vi "SDT_WriteFileDecayCurves.vi"(4 "adc_re[dig]":i16=256, 5 "ActiveModule":string[](array[string]), 6 "EndTimeArray":dbl[](array[numeric]), 7 "DecayMatrix":u32[][](array[numeric]), 8 "ErrorIn":errorcluster, 9 "SPCdata":T13[](array[typedef]) {"scan_flyback" format="%x"}, 10 "FileType":T1=2 items=["non-Fifo"=1, "Fifo"=2, "FifoImage"=3], 11 "SDT-FilePath":path=path "\\\\lab13\\C/Users/jannis/Desktop/ZeissFifo.sdt") -> (0 "ErrorOut":errorcluster)   [LabVIEW 2019]
doc: "This VI writes a SDT-file to disc. The SetUp and the MeasureInfo blocks are created and appended with the data blocks. \nThis VI is limited to writing a DecayMatrix from a FIFO-Image recording and optional an IntensityImage to file. For single mode recordings use the spcmdll VI \\Public\\Configure\\Memory Transfer\\SPC_save_data_to_sdtfile.vi.\nFor a description of the format for the Data input cluster to this VI see the usage in \\Example\\ImagingEventStream-SimpleFifoImage.vi. Leave either of the cluster input arrays empty to not save them to disc.\nFor a description of the *.sdt file format see: SPC_data_file_structure.h\n\ninfo@becker-hickl.com"
uses:
  SPC_Controls/bhfile_header.ctl
  SPC_Controls/SPCdata.ctl
  SPC_Controls/MeasureInfo_PartB.ctl
  SPC_Controls/MeasStopInfo.ctl
  SPC_Controls/MeasFCSInfo.ctl
  SPC_Controls/MeasureInfo_PartE.ctl
  SPC_Controls/MeasHISTInfo.ctl
  SPC_Controls/HISTInfoExt.ctl
  SPC_Controls/MeasureInfo_PartI.ctl
  SPC_Controls/MeasureInfo_PartK.ctl
  SPC_Controls/MeasureInfo_PartM.ctl
  SPC_Controls/MeasureInfo.ctl
  SPC_Controls/BHFileBlockHeader.ctl
  SPC_Controls/FileType.ctl
panel:
  out "Info Block":string
  out "BHFileBlockHeaders":T2[](array[typedef])
  out "MeasureInfos":T3[](array[typedef]) {"MeasFCSInfo"."end_time" format="%#_7g"; "MeasStopInfo"."flags" format="x%x"}
  out "BlockLengths":i32[](array[numeric])
  out "bhfile_header":T14 {"chksum" format="x%x"; "header_valid" format="x%x"}
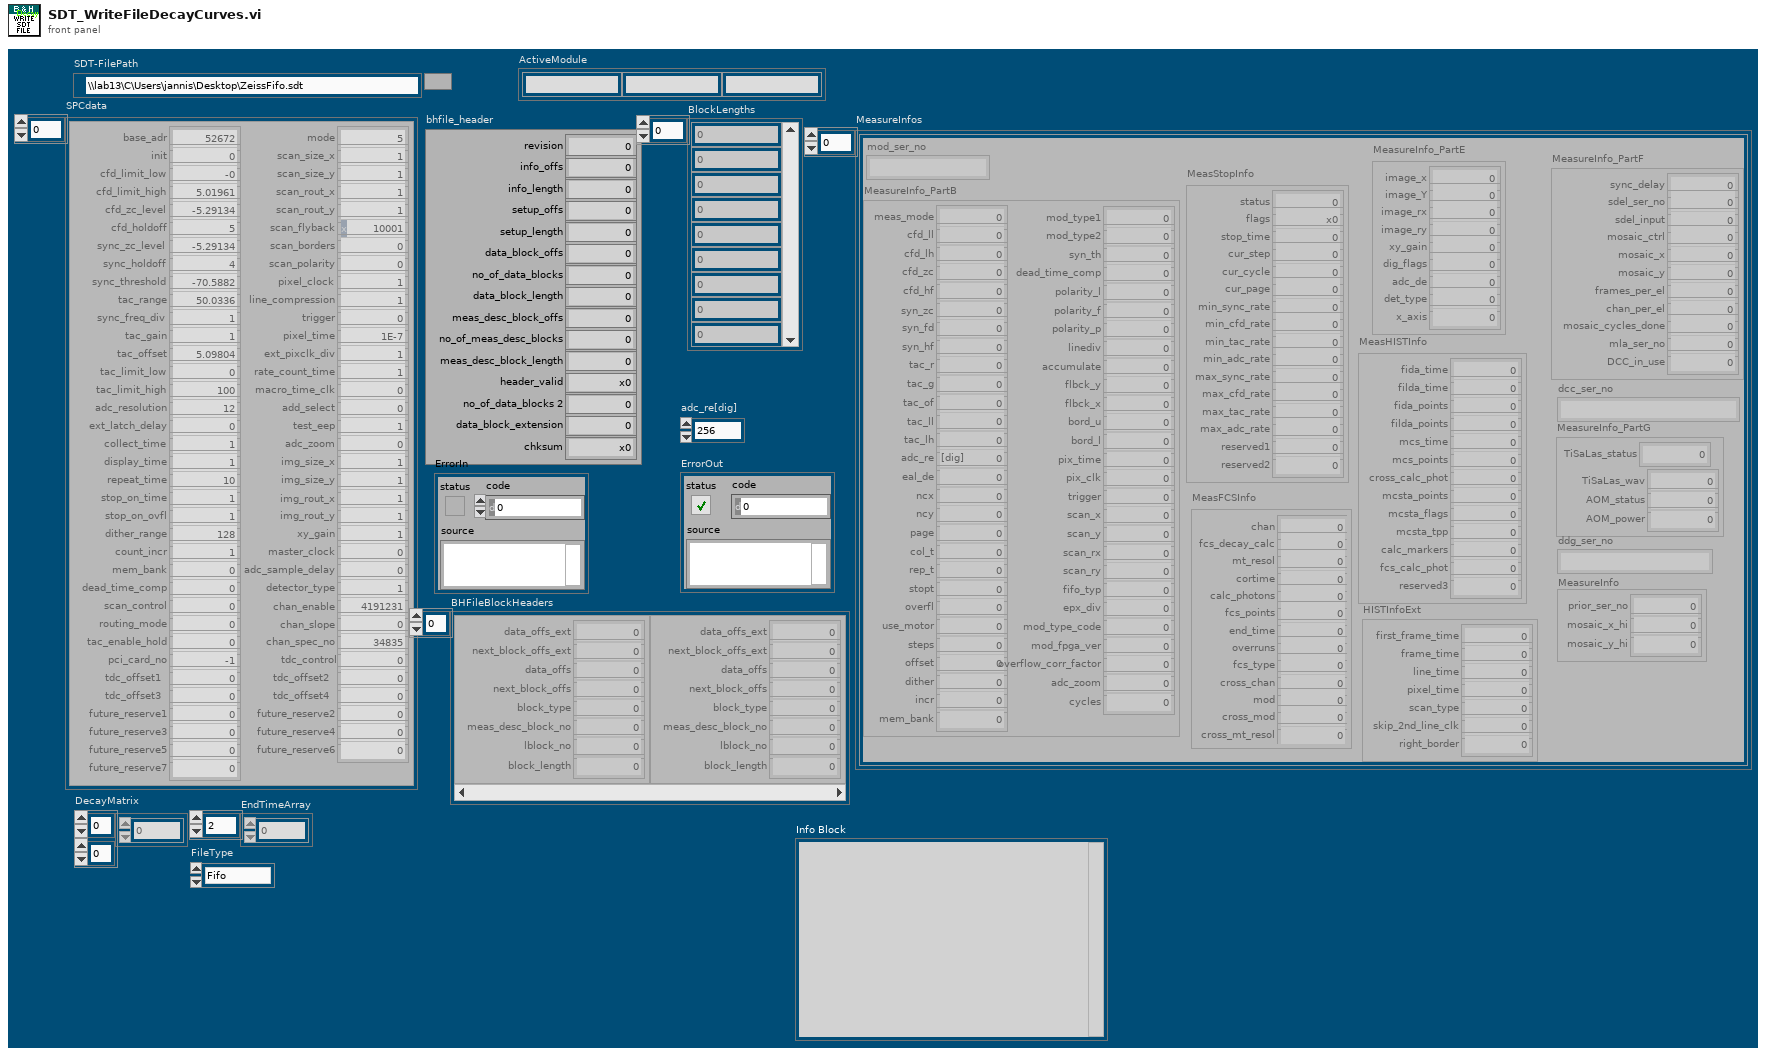
[diagram p1: front panel]
types:
  T1 = typedef "FileType.ctl" = u16
  T2 = typedef "BHFileBlockHeader.ctl" = cluster{"data_offs_ext":u8, "next_block_offs_ext":u8, "data_offs":u32, "next_block_offs":u32, "block_type":u16, "meas_desc_block_no":i16, "lblock_no":u32, "block_length":u32}
  T3 = typedef "MeasureInfo.ctl" = cluster{"mod_ser_no":string, "MeasureInfo_PartB":T4, "MeasStopInfo":T5, "MeasFCSInfo":T6, "MeasureInfo_PartE":T7, "MeasHISTInfo":T8, "HISTInfoExt":T9, "MeasureInfo_PartF":T10, "dcc_ser_no":string, "MeasureInfo_PartG":T11, "ddg_ser_no":string, "MeasureInfo":T12}
  T4 = typedef "MeasureInfo_PartB.ctl" = cluster{"meas_mode":i16, "cfd_ll":sgl, "cfd_lh":sgl, "cfd_zc":sgl, "cfd_hf":sgl, "syn_zc":sgl, "syn_fd":i16, "syn_hf":sgl, "tac_r":sgl, "tac_g":i16, "tac_of":sgl, "tac_ll":sgl, "tac_lh":sgl, "adc_re":i16, "eal_de":i16, "ncx":i16, "ncy":i16, "page":u16, "col_t":sgl, "rep_t":sgl, "stopt":i16, "overfl":i8, "use_motor":i16, "steps":u16, "offset":sgl, "dither":i16, "incr":i16, "mem_bank":i16, "mod_type1":u64, "mod_type2":u64, "syn_th":sgl, "dead_time_comp":i16, "polarity_l":i16, "polarity_f":i16, "polarity_p":i16, "linediv":i16, "accumulate":i16, "flbck_y":i32, "flbck_x":i32, "bord_u":i32, "bord_l":i32, "pix_time":sgl, "pix_clk":i16, "trigger":i16, "scan_x":i32, "scan_y":i32, "scan_rx":i32, "scan_ry":i32, "fifo_typ":i16, "epx_div":i32, "mod_type_code":u16, "mod_fpga_ver":u16, "overflow_corr_factor":sgl, "adc_zoom":i32, "cycles":i32}
  T5 = typedef "MeasStopInfo.ctl" = cluster{"status":u16, "flags":u16, "stop_time":sgl, "cur_step":i32, "cur_cycle":i32, "cur_page":i32, "min_sync_rate":sgl, "min_cfd_rate":sgl, "min_tac_rate":sgl, "min_adc_rate":sgl, "max_sync_rate":sgl, "max_cfd_rate":sgl, "max_tac_rate":sgl, "max_adc_rate":sgl, "reserved1":i32, "reserved2":sgl}
  T6 = typedef "MeasFCSInfo.ctl" = cluster{"chan":u16, "fcs_decay_calc":u16, "mt_resol":u32, "cortime":sgl, "calc_photons":u32, "fcs_points":i32, "end_time":sgl, "overruns":u16, "fcs_type":u16, "cross_chan":u16, "mod":u16, "cross_mod":u16, "cross_mt_resol":u32}
  T7 = typedef "MeasureInfo_PartE.ctl" = cluster{"image_x":i32, "image_Y":i32, "image_rx":i32, "image_ry":i32, "xy_gain":i16, "dig_flags":i16, "adc_de":i16, "det_type":i16, "x_axis":i16}
  T8 = typedef "MeasHISTInfo.ctl" = cluster{"fida_time":sgl, "filda_time":sgl, "fida_points":i32, "filda_points":i32, "mcs_time":sgl, "mcs_points":i32, "cross_calc_phot":u32, "mcsta_points":u16, "mcsta_flags":u16, "mcsta_tpp":u32, "calc_markers":u32, "fcs_calc_phot":u32, "reserved3":u32}
  T9 = typedef "HISTInfoExt.ctl" = cluster{"first_frame_time":sgl, "frame_time":sgl, "line_time":sgl, "pixel_time":sgl, "scan_type":i16, "skip_2nd_line_clk":i16, "right_border":u32}
  T10 = typedef "MeasureInfo_PartI.ctl" = cluster{"sync_delay":sgl, "sdel_ser_no":u16, "sdel_input":i8, "mosaic_ctrl":i8, "mosaic_x":u8, "mosaic_y":u8, "frames_per_el":i16, "chan_per_el":i16, "mosaic_cycles_done":i32, "mla_ser_no":u16, "DCC_in_use":u8}
  T11 = typedef "MeasureInfo_PartK.ctl" = cluster{"TiSaLas_status":u16, "TiSaLas_wav":u16, "AOM_status":u8, "AOM_power":u8}
  T12 = typedef "MeasureInfo_PartM.ctl" = cluster{"prior_ser_no":i32, "mosaic_x_hi":u8, "mosaic_y_hi":u8}
  T13 = typedef "SPCdata.ctl" = cluster{"base_adr":u16, "init":i16, "cfd_limit_low":sgl, "cfd_limit_high":sgl, "cfd_zc_level":sgl, "cfd_holdoff":sgl, "sync_zc_level":sgl, "sync_holdoff":sgl, "sync_threshold":sgl, "tac_range":sgl, "sync_freq_div":i16, "tac_gain":i16, "tac_offset":sgl, "tac_limit_low":sgl, "tac_limit_high":sgl, "adc_resolution":i16, "ext_latch_delay":i16, "collect_time":sgl, "display_time":sgl, "repeat_time":sgl, "stop_on_time":i16, "stop_on_ovfl":i16, "dither_range":i16, "count_incr":i16, "mem_bank":i16, "dead_time_comp":i16, "scan_control":u16, "routing_mode":u16, "tac_enable_hold":sgl, "pci_card_no":i16, "mode":u16, "scan_size_x":u32, "scan_size_y":u32, "scan_rout_x":u32, "scan_rout_y":u32, "scan_flyback":u32, "scan_borders":u32, "scan_polarity":u16, "pixel_clock":u16, "line_compression":u16, "trigger":u16, "pixel_time":sgl, "ext_pixclk_div":u32, "rate_count_time":sgl, "macro_time_clk":i16, "add_select":i16, "test_eep":i16, "adc_zoom":i16, "img_size_x":u32, "img_size_y":u32, "img_rout_x":u32, "img_rout_y":u32, "xy_gain":i16, "master_clock":i16, "adc_sample_delay":i16, "detector_type":i16, "chan_enable":u32, "chan_slope":u32, "chan_spec_no":u32, "tdc_control":u32, "tdc_offset1":sgl, "tdc_offset2":sgl, "tdc_offset3":sgl, "tdc_offset4":sgl, "future_reserve1":u64, "future_reserve2":u64, "future_reserve3":u64, "future_reserve4":u64, "future_reserve5":u64, "future_reserve6":u64, "future_reserve7":u64}
  T14 = typedef "bhfile_header.ctl" = cluster{"revision":i16, "info_offs":i32, "info_length":i16, "setup_offs":i32, "setup_length":u16, "data_block_offs":i32, "no_of_data_blocks":i16, "data_block_length":u32, "meas_desc_block_offs":i32, "no_of_meas_desc_blocks":i16, "meas_desc_block_length":i16, "header_valid":u16, "no_of_data_blocks 2":u32, "data_block_extension":u16, "chksum":u16}
  T15 = enum16{"open", "replace", "create", "open or create", "replace or create", "replace or create with confirmation"}
  T16 = enum16{"big-endian, network order", "native, host order", "little-endian"}
  T17 = typedef "BHModuleType.ctl" = i16
  T18 = typedef "ModuleType.ctl" = i16
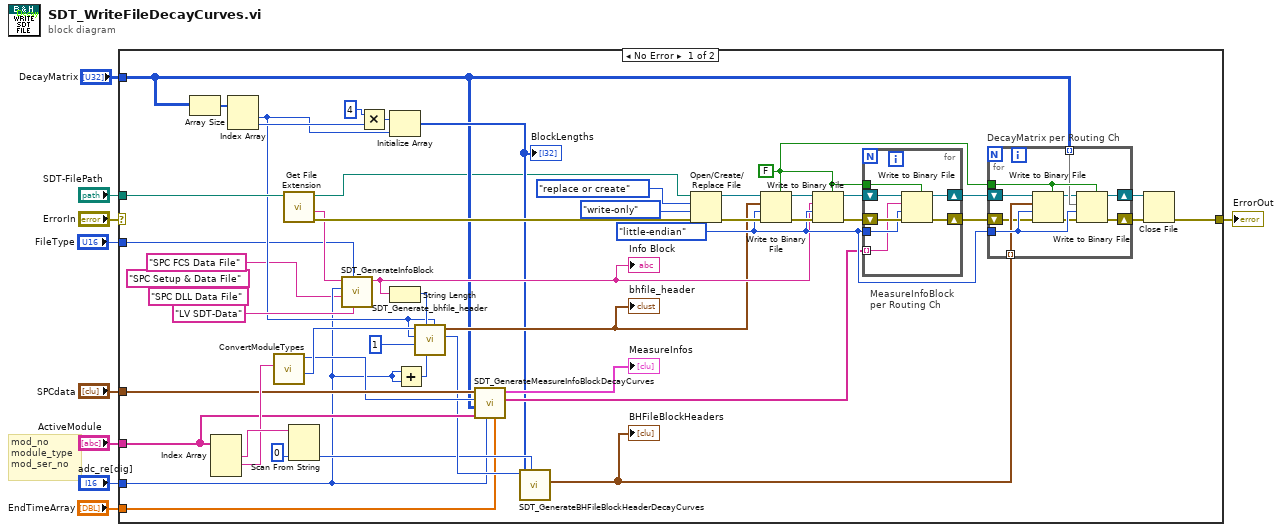
[diagram p0: block diagram]
diagram:
  # "mod_no\nmodule_type\nmod_ser_no"
  n1 = case shown="No Error" "ErrorIn" {
    selector: "ErrorIn" -> [_ w75]
    tunnel: [w10 w75] -> w8
    tunnel: "SPCdata" -> [w32 _]
    tunnel: "ActiveModule" -> [w30 _]
    tunnel: "SDT-FilePath" -> [w24 _]
    tunnel: "DecayMatrix" -> [w21 _]
    tunnel: "adc_re[dig]" -> [w16 _]
    tunnel: "EndTimeArray" -> [w13 _]
    tunnel: "FileType" -> [w12 _]
    frame No Error {
      (unwired) "SPC Setup & Data File" ("FileID")
      (unwired) "SPC DLL Data File" ("FileID")
      w48 = FALSE ("prepend array or string size? (T)")
      w47 = T16."little-endian" ("byte order (0:big-endian, network order)")
      n2 = Array Size(array=w21) -> (size(s)=w40:i32[])
      n3 = Index Array(array=w30) -> (element #1=w44:string, element #2=w41:string)  [unwired: 3 in, 1 out]
      n4 = Index Array(array=w40) -> (element #1=w18:i32, element #2=w20:i32)  [unwired: 2 in]
      n5 = call "ConvertModuleTypes.vi"("ModuleTypeStringIn"=w41) -> ("BHModuleType"=w33:T17, "Module TypeOut"=w31:T18)  [unwired: 8 in, 1 out]
      n6 = call <vilib>:"Get File Extension.vi"("file"=w24) -> ("error out"=w52:errorcluster, "filename without extension"=w37:string, "dup file"=w11:path)  [unwired: 6 in, 2 out]
      n7 = Scan From String(input string=w44, default 1=u32 0 ("meas_desc_block_no")) -> (output 1=w25:u32)  [unwired: 3 in, 3 out]
      n8 = call "SDT_GenerateInfoBlock.vi"("Contents"="LV SDT-Data", "FileType"=w12, "FileID"="SPC FCS Data File", "adc_re[dig]"=w16, "FilenameNoExtension"=w37) -> ("Info Block"=w35:string)  [unwired: 6 in]
      "Info Block" <- w35
      n9 = Multiply(x=4 ("y"), y=w20) -> (x*y=w19:i32)
      n10 = Initialize Array(w19, w18) -> (w22:i32[])
      "BlockLengths" <- w22
      n11 = String Length(string=w35) -> (length=w34:i32)
      n12 = Add(x=w16, y=w16) -> (x+y=w15:i16)
      n13 = call "SDT_Generate_bhfile_header.vi"("no_of_data_blocks"=w18, "adc_re[dig]"=w15, "info_length"=w34, "ImageSize"=u32 1, "NoOfRoutingChannel"=w18, "BHModuleType"=w33) -> ("data_block_offs"=w26:i32, "bhfile_header"=w28:T14)  [unwired: 4 in]
      "bhfile_header" <- w28
      n14 = call "SDT_GenerateMeasureInfoBlockDecayCurves.vi"("EndTimeArray"=w13, "adc_re[dig]"=w16, "ActiveModule"=w30, "DecayMatrix"=w21, "Module Type"=w31, "SPCdata"=w32) -> ("MeasureInfoStrings"=w23:string[], "MeasureInfos"=→"MeasureInfos":T3[])  [unwired: 4 in]
      n15 = call "SDT_GenerateBHFileBlockHeaderDecayCurves.vi"("ModuleNo"=w25, "BlockLengths"=w22, "data_block_offs"=w26) -> ("BHFileBlockHeaders"=w27:T2[])  [unwired: 7 in, 1 out]
      "BHFileBlockHeaders" <- w27
      n16 = Open/Create/Replace File(file path (use dialog)=w11, error in=w52, operation (0:open)=T15."replace or create", access (0:read/write)=enum16{"read/write", "read-only", "write-only"}."write-only") -> (refnum out=w55:refnum<file>, error out=w51:errorcluster)  [unwired: 2 in, 1 out]
      n17 = Write to Binary File(file (use dialog)=w55, data=w28, error in=w51, 5:w48, 9:w47) -> (refnum out=w54:refnum<file>, error out=w50:errorcluster)  [unwired: 1 in, 1 out]
      n18 = Write to Binary File(file (use dialog)=w54, data=w35, error in=w50, 5:w48, 9:w47) -> (refnum out=w53:refnum<file>, error out=w49:errorcluster)  [unwired: 1 in, 1 out]
      n19 = for "MeasureInfoBlock\nper Routing Ch" {
        tunnel: w48 -> [w62]
        tunnel: w47 -> [w61]
        shift-right: [w60] -> w39
        shift-left: w53 -> [w64]
        shift-right: [w59] -> w38
        shift-left: w49 -> [w63]
        tunnel: w23 -> [w58] mode=indexing
        n20 = Write to Binary File(file (use dialog)=w64, data=w58, error in=w63, 5:w62, 9:w61) -> (refnum out=w60:refnum<file>, error out=w59:errorcluster)  [unwired: 1 in, 1 out]
      }
      n21 = for "DecayMatrix per Routing Ch" {
        tunnel: w48 -> [w74]
        tunnel: w47 -> [w73]
        tunnel: w27 -> [w70] mode=indexing
        tunnel: w21 -> [w69] mode=indexing
        shift-right: [w71] -> w45
        shift-left: w39 -> [w68]
        shift-right: [w72] -> w46
        shift-left: w38 -> [w67]
        n22 = Write to Binary File(file (use dialog)=w68, data=w70, error in=w67, 5:w74, 9:w73) -> (refnum out=w66:refnum<file>, error out=w65:errorcluster)  [unwired: 1 in, 1 out]
        n23 = Write to Binary File(file (use dialog)=w66, data=w69, error in=w65, 5:w74, 9:w73) -> (refnum out=w71:refnum<file>, error out=w72:errorcluster)  [unwired: 1 in, 1 out]
      }
      n24 = Close File(refnum=w45, error in=w46) -> (error out=w10:errorcluster)  [unwired: 1 out]
    }
    frame Error {
    }
  }
  "ErrorOut" <- w8
